vi "Close Front Panel.vi"(8 "error in (no error)":errorcluster, 11 "VI File Path":path) -> (0 "error out":errorcluster)   [LabVIEW 2024]
doc: "Closes the front panel of a VI."
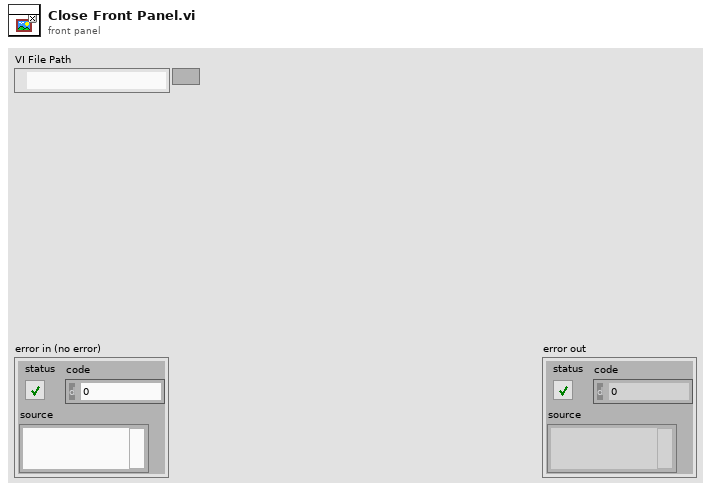
[diagram p1: front panel]
types:
  T1 = enum32{"Invalid", "Standard", "Closed", "Hidden", "Minimized", "Maximized"}
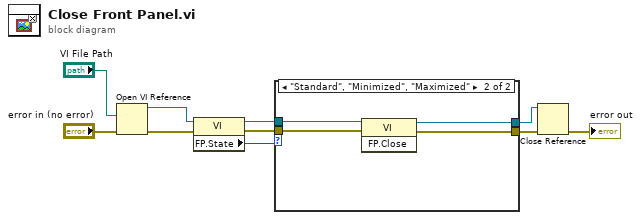
[diagram p0: block diagram]
diagram:
  n1 = Open VI Reference(vi path="VI File Path", error in (no error)="error in (no error)") -> (vi reference=w5:refnum<vi>, error out=w4:errorcluster)  [unwired: 4 in]
  n2 = property class="VI"(reference=w5, error in=w4) -> (reference out=w2:refnum<vi>, error out=w3:errorcluster, "FP.State"=w1:T1)
  n3 = case shown="\"Standard\", \"Minimized\", \"Maximized\"" w1 {
    tunnel: [w12 w16] -> w7
    tunnel: [w11 w15] -> w6
    tunnel: w3 -> [w12 w14]
    tunnel: w2 -> [w11 w13]
    frame "Invalid", "Closed", "Hidden", Default {
    }
    frame "Standard", "Minimized", "Maximized" {
      n4 = invoke class="VI" method="FP.Close"(reference=w13, error in=w14) -> (reference out=w15:refnum<vi>, error out=w16:errorcluster)  [unwired: 1 in, 1 out]
    }
  }
  n5 = Close Reference(reference=w6, error in (no error)=w7) -> (error out=→"error out":errorcluster)
